vi "DmgrFreeDvcEnum.vi"(8 "Error In":errorcluster) -> (0 "Error Out":errorcluster)   [LabVIEW 2011, in "LVH-Adept.lvlib" / "DMGR.lvlib"]
doc: "Free Enumerated Devices"
uses:
  DMGR.lvlib
  <vilib>/LabVIEW Hacker/Adept/Private/Resources/dmgr.dll
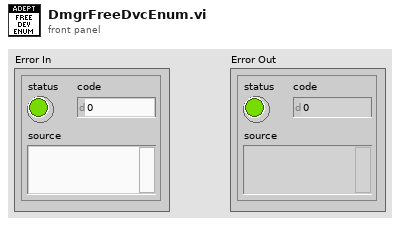
[diagram p1: front panel]
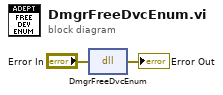
[diagram p0: block diagram]
diagram:
  n1 = dll-call lib="C:/Program Files (x86)/National Instruments/LabVIEW 2011/vi.lib/LabVIEW Hacker/Adept/Private/Resources/dmgr.dll" fn="DmgrFreeDvcEnum"(error in="Error In") -> (error out=→"Error Out":errorcluster)  [unwired: 3 in, 1 out]
